vi "Add reading.vi"(7 "Power (mW)":dbl, 8 "error in (no error)":errorcluster, 9 "Width (GHz)":dbl, 10 "Frequency (GHz)":dbl, 11 "Power control in":refnum<class "Power control.lvclass">) -> (0 "error out":errorcluster, 3 "Power control out":refnum<class "Power control.lvclass">)   [LabVIEW 2019, in "Power control.lvclass"]
uses:
  Power control.lvclass
  Power control.lvclass/Power control.ctl
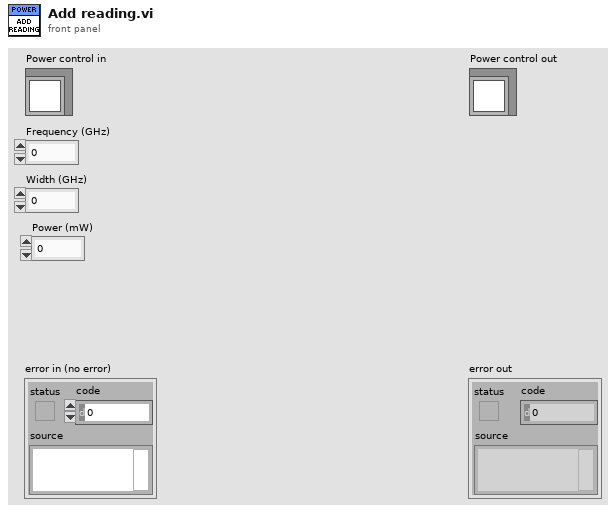
[diagram p1: front panel]
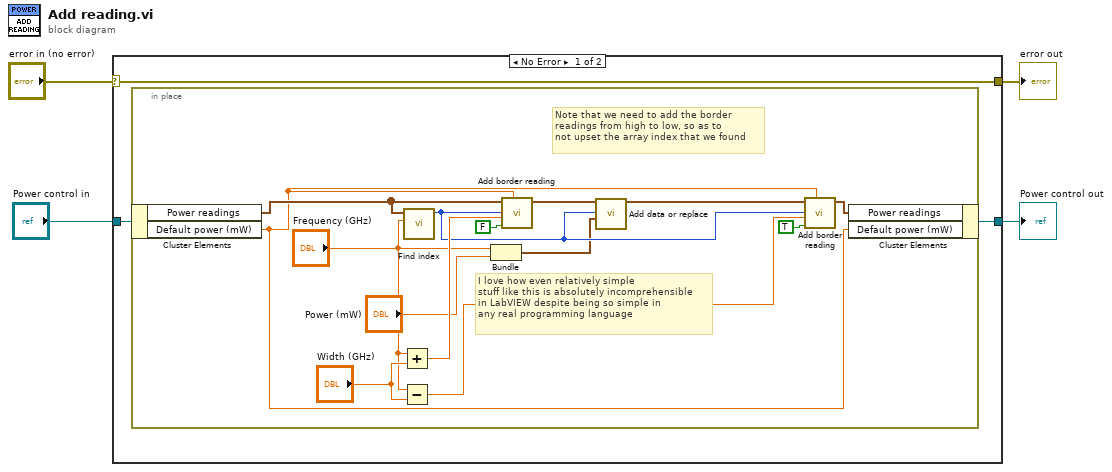
[diagram p0: block diagram]
diagram:
  n1 = case shown="No Error" "error in (no error)" {
    selector: "error in (no error)" -> [w7 w23]
    tunnel: [w7 w23] -> w3
    tunnel: [w5 w22] -> w1
    tunnel: "Power control in" -> [w6 w22]
    frame No Error {
      n2 = in-place {
        # "I love how even relatively simple\nstuff like this is absolutely incomprehensible\nin LabVIEW despite being so simple in\nany real programming language"
        # "Note that we need to add the border\nreadings from high to low, so as to\nnot upset the array index that we found"
        n3 = in-place-cluster #1(w6) -> ("Power readings"=w19:cluster{"Frequency":dbl, "Power":dbl}[], "Default power (mW)"=w8:dbl)
        n4 = Add(x="Frequency (GHz)", y="Width (GHz)") -> (x+y=w17:dbl)
        n5 = Subtract(x="Frequency (GHz)", y="Width (GHz)") -> (x-y=w21:dbl)
        n6 = call "Find index.vi"("Frequency (GHz)"="Frequency (GHz)", "Power readings"=w19) -> ("Index of matching or greater point"=w13:i32)  [unwired: 9 in]
        n7 = Bundle("Frequency (GHz)"="Frequency (GHz)", "Power (mW)"="Power (mW)") -> (w10:cluster{"Frequency (GHz)":dbl, "Power (mW)":dbl})  [unwired: 1 in]
        n8 = call "Add border reading.vi"("Default power"=w8, "Lower border?"=FALSE, "Border frequency"=w17, "Border index"=w13, "Power readings in"=w19) -> ("Power readings out"=w15:cluster{"Frequency":dbl, "Power":dbl}[])  [unwired: 6 in]
        n9 = call "Add data or replace.vi"("Power data"=w10, "Index"=w13, "Power readings in"=w15) -> ("Power readings out"=w14:cluster{"Frequency":dbl, "Power":dbl}[])  [unwired: 8 in]
        n10 = call "Add border reading.vi"("Default power"=w8, "Lower border?"=TRUE, "Border frequency"=w21, "Border index"=w13, "Power readings in"=w14) -> ("Power readings out"=w9:cluster{"Frequency":dbl, "Power":dbl}[])  [unwired: 6 in]
        n11 = in-place-cluster #1("Power readings"=w9, "Default power (mW)"=w8) -> (w5:refnum<class "Power control.lvclass">)
      }
    }
    frame Error {
    }
  }
  "error out" <- w3
  "Power control out" <- w1
